vi "量测站data内容.vi"() -> (0 "tablename":string, 3 "data":string[](array[string]))   [LabVIEW 2017]
uses:
  Sqlite/CBB/ReadAllData.vi
  Sqlite/SQLite.lvlib
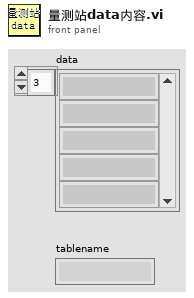
[diagram p1: front panel]
types:
  T1 = typedef "缓存操作选项.ctl" = enum16{"初始化", "量测缓存写入", "前侧获取索引", "后侧获取索引", "前侧更新索引", "后侧更新索引", "获取寄存器"}
  T2 = typedef "交互选项.ctl" = enum16{"初始化", "寄存器提取", "更新单点量测值", "更新单侧到对应动子集合", "动子1&2执行完删除缓存", "动子3&4执行完删除缓存"}
  T3 = typedef "laser模组选项.ctl" = enum16{"初始化", "提取3D值", "寄存器提取"}
  T4 = typedef "barcode流程.ctl" = enum16{"串口初始化", "发指令打开刷枪", "等待获取OK信号", "获取寄存器"}
  T5 = typedef "pathcheck选项.ctl" = enum16{"ProductData", "CTData", "ERData", "IOTDATA"}
  T6 = typedef "单点提取集合.ctl" = cluster{"筛选信息":T7, "提取status":T10, "厚度信息":T11}
  T7 = typedef "筛选信息.ctl" = cluster{"模组编号":T8, "抓手编号":T9, "标签机编号":T9, "贴合点位":u32}
  T8 = typedef "手动执行模组信息.ctl" = enum16{"动子1模组", "动子2模组", "动子3模组", "动子4模组"}
  T9 = typedef "抓手OR标签机.ctl" = enum16{"编号1", "编号2", "编号3"}
  T10 = typedef "提取status.ctl" = enum16{"标签机匹配OK", "无需贴合", "无对应的标签机", "标签机维护信息有误"}
  T11 = typedef "厚度信息.ctl" = cluster{"chassis厚度":dbl, "trackpad厚度":dbl, "shim厚度":dbl, "shim规格":dbl}
  T12 = typedef "Laser Measure Data集合.ctl" = cluster{"Chassis Laser Measure Data":T13[], "Magnet Laser Measure Data":T13[]}
  T13 = typedef "step数据.ctl" = cluster{"数据":string, "状态":bool}
  T14 = cluster{"chassis厚度":string, "trackpad厚度":string, "shim厚度":string, "shim规格":string}
  T15 = typedef "barcode结果显示.ctl" = cluster{"scanok?":bool, "barcode":string, "Time":dbl}
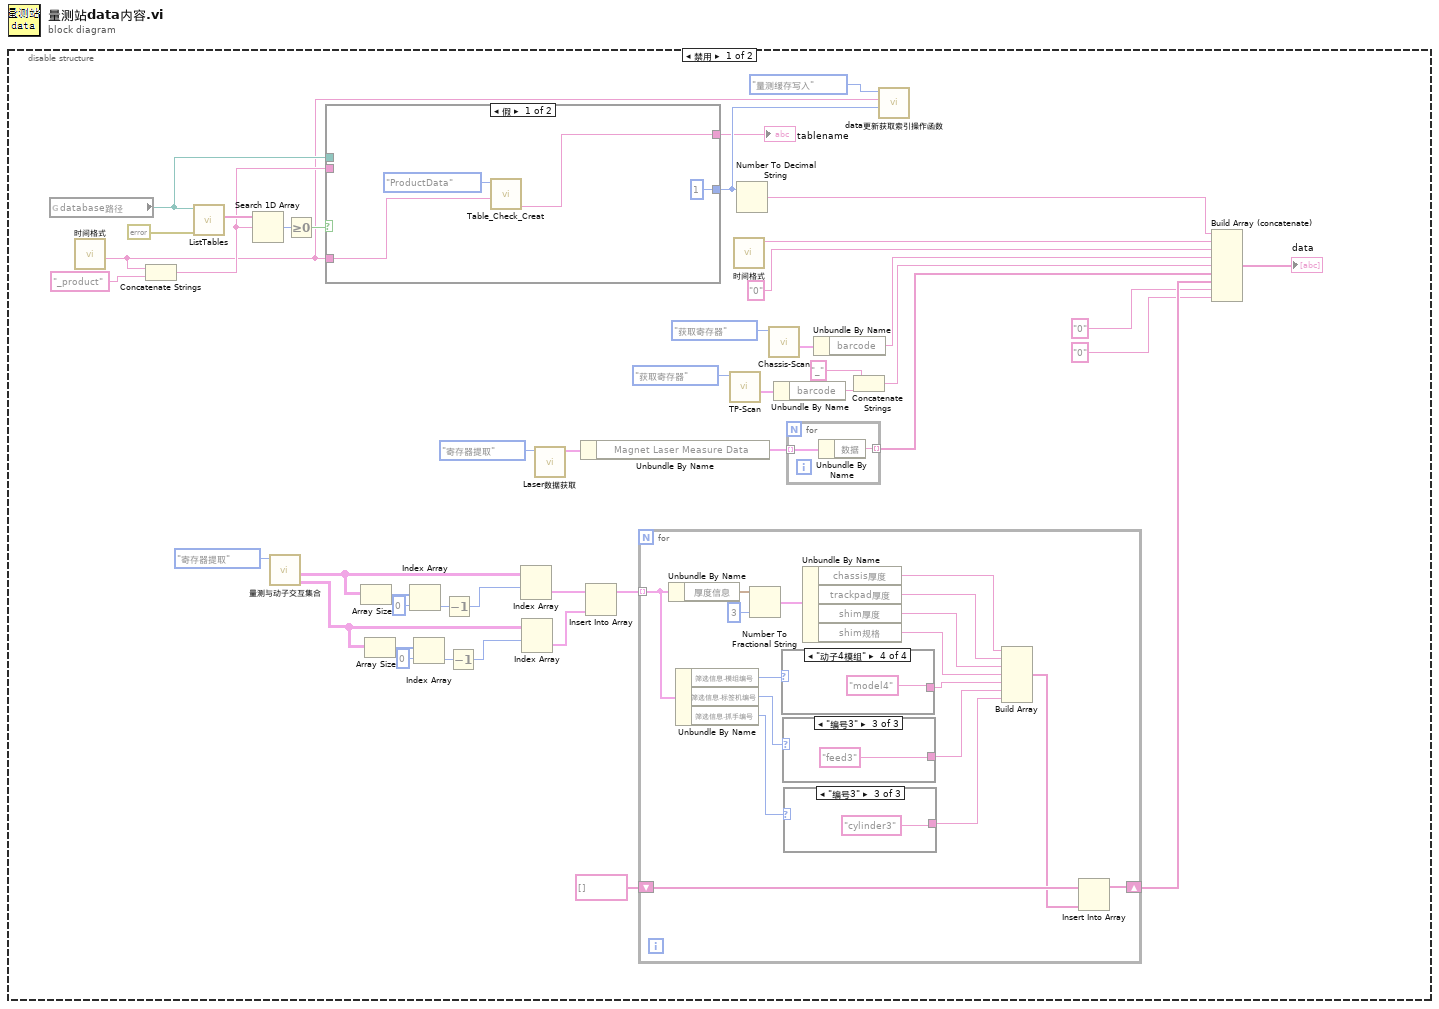
[diagram p0: block diagram]
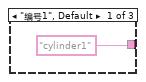
[diagram p2: hidden frame]
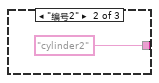
[diagram p3: hidden frame]
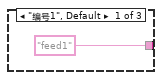
[diagram p4: hidden frame]
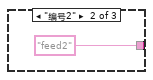
[diagram p5: hidden frame]
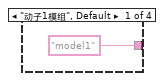
[diagram p6: hidden frame]
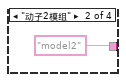
[diagram p7: hidden frame]
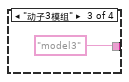
[diagram p8: hidden frame]
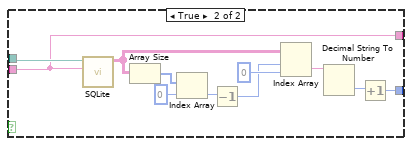
[diagram p9: hidden frame]
diagram:
  n1 = disable-structure shown="禁用" {
    frame Disabled {
      n2 = global read "数据库全局.vi" "database路径"() -> (w4:path)
      n3 = call "时间格式.vi"() -> ("_Date"=w2:string)  [unwired: 7 in, 4 out]
      n4 = Concatenate Strings(w2, "_product" ("字符串")) -> (w3:string)
      n5 = call "ListTables.vi"("error in (no error)"=errorcluster {"status"=FALSE, "code"=0, "source"=""}, "DbPath"=w4) -> ("Tables"=w8:string[])  [unwired: 6 in, 3 out]
      n6 = Search 1D Array(1D array=w8, element=w3) -> (index of element=w9:i32)  [unwired: 1 in]
      n7 = call "量测与动子交互集合.vi"("交互选项"=交互选项."寄存器提取") -> ("动子3&4侧输出"=w26:T6[][], "动子1&2侧输出"=w35:T6[][])  [unwired: 8 in, 1 out]
      n8 = Greater Or Equal To 0?(x=w9) -> (x >= 0?=w5:bool)
      n9 = case shown="假" w5 {
        tunnel: w4 -> [_ w89]
        tunnel: w3 -> [_ w79]
        tunnel: [1 w80] -> w10
        tunnel: w2 -> [w76 _]
        tunnel: [w75 w79] -> w1
        frame False {
          n10 = call "Table_Check_Creat.vi"("_datetime"=w76, "pathcheck选项"=pathcheck选项."ProductData") -> ("tablename"=w75:string)  [unwired: 7 in, 2 out]
        }
        frame True {
          n11 = call-poly "SQLite.vi"("Table Name"=w79, "DbPath"=w89) -> ("Results"=w87:string[][])  [unwired: 4 in, 5 out]
          n12 = Array Size(array=w87) -> (size(s)=w86:i32[])
          n13 = Index Array(array=w86, index=0 ("索引")) -> (element=w84:i32)
          n14 = Decrement(x=w84) -> (x-1=w83:i32)
          n15 = Index Array(array=w87, index (row)=w83, index (col)=0 ("禁用的索引 (列)")) -> (element=w82:string)
          n16 = Decimal String To Number(string=w82) -> (number=w81:i32)  [unwired: 2 in, 1 out]
          n17 = Increment(x=w81) -> (x+1=w80:i32)
        }
      }
      "tablename" <- w1
      n18 = Array Size(array=w35) -> (size(s)=w34:i32[])
      n19 = Array Size(array=w26) -> (size(s)=w27:i32[])
      n20 = Index Array(array=w34, index=0 ("索引")) -> (element=w32:i32)
      n21 = Index Array(array=w27, index=0 ("索引")) -> (element=w29:i32)
      n22 = Decrement(x=w32) -> (x-1=w31:i32)
      n23 = Decrement(x=w29) -> (x-1=w30:i32)
      n24 = Index Array(array=w35, index (row)=w31) -> (element=w25:T6[])  [unwired: 1 in]
      n25 = Index Array(array=w26, index (row)=w30) -> (element=w24:T6[])  [unwired: 1 in]
      n26 = call "Laser数据获取.vi"("laser模组选项"=laser模组选项."寄存器提取") -> ("Laser Measure Data集合"=w39:T12)  [unwired: 7 in, 3 out]
      n27 = Unbundle By Name(w39) -> ("Magnet Laser Measure Data"=w38:T13[])
      n28 = Insert Into Array(array=w25, new element=w24) -> (w23:T6[])  [unwired: 1 in]
      n29 = for {
        tunnel: w23 -> [w59] mode=indexing
        shift-right: [w50] -> w21
        shift-left: string[] [] -> [w52]
        n30 = Unbundle By Name(w59) -> ("厚度信息"=w62:T11)
        n31 = Unbundle By Name(w59) -> ("筛选信息.模组编号"=w58:T8, "筛选信息.标签机编号"=w57:T9, "筛选信息.抓手编号"=w56:T9)
        n32 = Number To Fractional String(number=w62, precision (6)=i16 3 ("精度(6)")) -> (F-format string=w60:T14)  [unwired: 2 in]
        n33 = case shown="\"动子4模组\"" w58 {
          tunnel: ["model1" "model2" "model3" "model4"] -> w48
          frame "动子1模组", Default {
          }
          frame "动子2模组" {
          }
          frame "动子3模组" {
          }
          frame "动子4模组" {
          }
        }
        n34 = case shown="\"编号3\"" w57 {
          tunnel: ["feed1" "feed2" "feed3"] -> w47
          frame "编号1", Default {
          }
          frame "编号2" {
          }
          frame "编号3" {
          }
        }
        n35 = case shown="\"编号3\"" w56 {
          tunnel: ["cylinder1" "cylinder2" "cylinder3"] -> w46
          frame "编号1", Default {
          }
          frame "编号2" {
          }
          frame "编号3" {
          }
        }
        n36 = Unbundle By Name(w60) -> ("chassis厚度"=w55:string, "trackpad厚度"=w54:string, "shim厚度"=w53:string, "shim规格"=w49:string)
        n37 = Build Array(w55, w54, w53, w49, w48, w47, w46) -> (w51:string[])
        n38 = Insert Into Array(array=w52, new element=w51) -> (w50:string[])  [unwired: 1 in]
      }
      n39 = call "TP-Scan.vi"("barcode流程"=barcode流程."获取寄存器") -> ("barcode结果显示"=w43:T15)  [unwired: 10 in]
      n40 = call "时间格式.vi"() -> ("日期/时间字符串"=w16:string)  [unwired: 7 in, 4 out]
      n41 = Number To Decimal String(number=w10) -> (decimal integer string=w17:string)  [unwired: 1 in]
      n42 = call "Chassis-Scan.vi"("barcode流程"=barcode流程."获取寄存器") -> ("barcode结果显示"=w42:T15)  [unwired: 10 in]
      n43 = Unbundle By Name(w43) -> ("barcode"=w20:string)
      n44 = for {
        tunnel: w38 -> [w74] mode=indexing
        tunnel: [w73] -> w36 mode=indexing
        n45 = Unbundle By Name(w74) -> ("数据"=w73:string)
      }
      n46 = Unbundle By Name(w42) -> ("barcode"=w41:string)
      n47 = Concatenate Strings("_" ("字符串"), w20) -> (w18:string)
      n48 = call "data更新获取索引操作函数.vi"("当前操作行"=w10, "当前_datetime"=w2, "缓存操作选项"=缓存操作选项."量测缓存写入") -> ()  [unwired: 7 in, 2 out]
      n49 = Build Array (concatenate)(w17, w16, "0", w41, w18, w36, w21, "0", "0") -> (→"data":string[])
    }
    frame Enabled {
    }
  }
